vi "Read Element of JSON Setups.vi"(8 "error in (no error)":errorcluster, 10 "index":u16, 11 "JSON in":refnum<class "JSON.lvclass">) -> (0 "error out":errorcluster, 2 "String":string, 3 "JSON out":refnum<class "JSON.lvclass">)   [LabVIEW 2018, in "JSON.lvclass"]
uses:
  JSON.lvclass
  JSON.lvclass/JSON.ctl
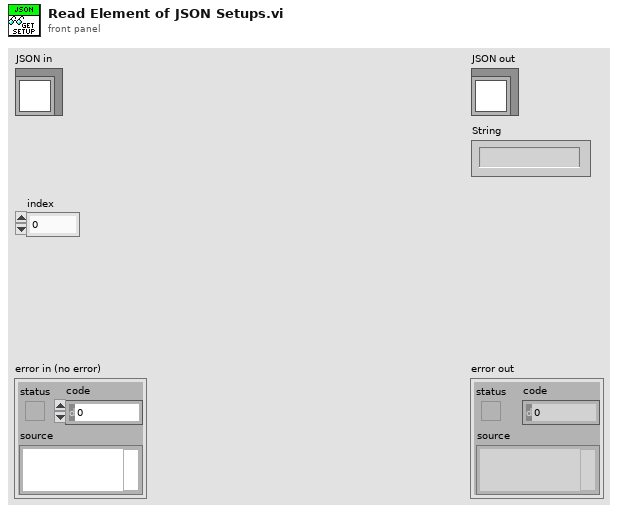
[diagram p1: front panel]
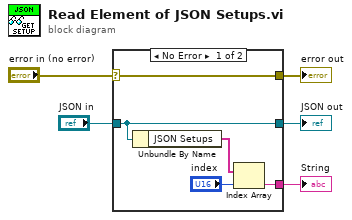
[diagram p0: block diagram]
diagram:
  n1 = case shown="No Error" "error in (no error)" {
    selector: "error in (no error)" -> [w10 w11]
    tunnel: [w10 w11] -> w4
    tunnel: [w9 w12] -> w2
    tunnel: "JSON in" -> [w9 w12]
    tunnel: [w7 _] -> w1
    frame No Error {
      n2 = Unbundle By Name(w9) -> ("JSON Setups"=w6:string[])
      n3 = Index Array(array=w6, index="index") -> (element=w7:string)
    }
    frame Error {
    }
  }
  "error out" <- w4
  "JSON out" <- w2
  "String" <- w1
